vi "Find Icon With Most Depth.vi"(0 "Icon Info":T1[](array[typedef])=[{"Width"=16, "Height"=16, "Depth"=8, "Resource Data"=[40, 0, 0, 0, 16, 0, 0, 0, 32, 0, 0, 0, 1, 0, 8, 0, 0, 0, 0, 0, 64, 1, 0, 0, 0, 0, 0, 0, 0, 0, 0, 0, 0, 0, 0, 0, 0, 0, 0, 0, 0, 0, 0, 0, 128, 0, 128, 0, 128, 0, 0, 0, 146, 126, 107, 0, 0, 128, 0, 0, 0, 128, 128, 0, 0, 0, 128, 0, 188, 165, 151, 0, 191, 174, 160, 0, 233, 207, 188, 0, 154, 130, 111, 0, 255, 0, 255, 0, 255, 0, 0, 0, 255, 255, 0, 0, 0, 255, 0, 0, 0, 255, 255, 0, 0, 0, 255, 0, 255, 255, 255, 0, 224, 241, 253, 0, 187, 167, 153, 0, 225, 242, 253, 0, 193, 229, 254, 0, 132, 204, 253, 0, 119, 198, 252, 0, 69, 157, 219, 0, 10, 153, 252, 0, 10, 153, 251, 0, 19, 156, 252, 0, 0, 122, 185, 0, 0, 98, 150, 0, 0, 74, 115, 0, 0, 50, 80, 0, 193, 228, 253, 0, 159, 214, 253, 0, 121, 198, 253, 0, 97, 189, 252, 0, 52, 170, 252, 0, 41, 165, 252, 0, 24, 159, 252, 0, 0, 73, 220, 0, 0, 61, 185, 0, 0, 49, 150, 0, 0, 37, 115, 0, 0, 25, 80, 0, 156, 214, 253, 0, 117, 197, 252, 0, 102, 191, 253, 0, 55, 171, 252, 0, 67, 155, 216, 0, 37, 37, 255, 0, 0, 0, 255, 0, 0, 0, 220, 0, 0, 0, 185, 0, 0, 0, 150, 0, 0, 0, 115, 0, 0, 0, 80, 0, 156, 213, 253, 0, 132, 203, 252, 0, 91, 186, 252, 0, 132, 202, 252, 0, 115, 72, 255, 0, 87, 37, 255, 0, 85, 0, 255, 0, 73, 0, 220, 0, 61, 0, 185, 0, 49, 0, 150, 0, 37, 0, 115, 0, 25, 0, 80, 0, 254, 252, 252, 0, 131, 202, 251, 0, 251, 245, 242, 0, 249, 242, 236, 0, 249, 241, 236, 0, 170, 37, 255, 0, 170, 0, 255, 0, 146, 0, 220, 0, 122, 0, 185, 0, 98, 0, 150, 0, 74, 0, 115, 0, 50, 0, 80, 0, 255, 254, 254, 0, 252, 248, 246, 0, 252, 246, 243, 0, 251, 244, 240, 0, 251, 245, 241, 0, 251, 244, 241, 0, 255, 0, 255, 0, 244, 229, 221, 0, 185, 0, 185, 0, 150, 0, 150, 0, 115, 0, 115, 0, 80, 0, 80, 0, 254, 252, 251, 0, 253, 249, 247, 0, 254, 251, 249, 0, 251, 244, 239, 0, 232, 208, 192, 0, 240, 223, 212, 0, 234, 212, 199, 0, 220, 0, 146, 0, 180, 157, 140, 0, 150, 0, 98, 0, 115, 0, 74, 0, 80, 0, 50, 0, 245, 236, 229, 0, 237, 220, 209, 0, 182, 159, 143, 0, 180, 157, 141, 0, 237, 216, 204, 0, 255, 37, 87, 0, 255, 0, 85, 0, 220, 0, 73, 0, 185, 0, 61, 0, 150, 0, 49, 0, 115, 0, 37, 0, 80, 0, 25, 0, 243, 231, 223, 0, 185, 168, 154, 0, 180, 156, 140, 0, 231, 207, 192, 0, 255, 72, 72, 0, 255, 37, 37, 0, 255, 0, 0, 0, 220, 0, 0, 0, 185, 0, 0, 0, 150, 0, 0, 0, 115, 0, 0, 0, 80, 0, 0, 0, 253, 250, 248, 0, 252, 248, 244, 0, 181, 157, 142, 0, 181, 158, 142, 0, 235, 214, 201, 0, 255, 87, 37, 0, 255, 85, 0, 0, 220, 73, 0, 0, 185, 61, 0, 0, 150, 49, 0, 0, 115, 37, 0, 0, 80, 25, 0, 0, 250, 241, 235, 0, 252, 248, 245, 0, 235, 216, 203, 0, 233, 212, 197, 0, 251, 243, 239, 0, 238, 219, 208, 0, 233, 211, 196, 0, 220, 146, 0, 0, 172, 150, 134, 0, 150, 98, 0, 0, 115, 74, 0, 0, 80, 50, 0, 0, 254, 254, 253, 0, 253, 250, 249, 0, 252, 249, 246, 0, 252, 247, 245, 0, 251, 245, 240, 0, 251, 246, 243, 0, 255, 255, 0, 0, 241, 226, 217, 0, 222, 191, 171, 0, 179, 155, 139, 0, 134, 115, 95, 0, 80, 80, 0, 0, 253, 252, 250, 0, 252, 247, 244, 0, 252, 246, 244, 0, 232, 208, 193, 0, 250, 242, 238, 0, 170, 255, 37, 0, 170, 255, 0, 0, 146, 220, 0, 0, 122, 185, 0, 0, 98, 150, 0, 0, 74, 115, 0, 0, 50, 80, 0, 0, 253, 251, 250, 0, 251, 246, 242, 0, 184, 167, 152, 0, 250, 241, 236, 0, 115, 255, 72, 0, 87, 255, 37, 0, 85, 255, 0, 0, 73, 220, 0, 0, 61, 185, 0, 0, 49, 150, 0, 0, 37, 115, 0, 0, 25, 80, 0, 0, 253, 250, 247, 0, 252, 246, 242, 0, 180, 157, 139, 0, 232, 208, 194, 0, 72, 255, 72, 0, 37, 255, 37, 0, 0, 255, 0, 0, 0, 220, 0, 0, 0, 185, 0, 0, 0, 150, 0, 0, 0, 115, 0, 0, 0, 80, 0, 0, 222, 241, 254, 0, 192, 226, 249, 0, 250, 243, 238, 0, 249, 240, 235, 0, 72, 255, 115, 0, 37, 255, 87, 0, 0, 255, 85, 0, 0, 220, 73, 0, 0, 185, 61, 0, 0, 150, 49, 0, 0, 115, 37, 0, 0, 80, 25, 0, 253, 251, 249, 0, 132, 202, 251, 0, 138, 206, 253, 0, 251, 242, 238, 0, 250, 242, 236, 0, 37, 255, 170, 0, 0, 255, 170, 0, 0, 220, 146, 0, 0, 185, 122, 0, 0, 150, 98, 0, 0, 115, 74, 0, 0, 80, 50, 0, 254, 253, 252, 0, 140, 207, 253, 0, 143, 208, 253, 0, 108, 193, 252, 0, 65, 175, 252, 0, 30, 161, 252, 0, 0, 255, 255, 0, 39, 164, 252, 0, 0, 185, 185, 0, 0, 150, 150, 0, 0, 115, 115, 0, 0, 80, 80, 0, 252, 242, 237, 0, 236, 229, 226, 0, 241, 226, 216, 0, 217, 205, 197, 0, 193, 173, 158, 0, 185, 164, 149, 0, 187, 168, 154, 0, 186, 166, 151, 0, 184, 162, 147, 0, 182, 160, 144, 0, 156, 134, 115, 0, 133, 108, 86, 0, 128, 109, 89, 0, 160, 139, 121, 0, 74, 74, 74, 0, 62, 62, 62, 0, 50, 50, 50, 0, 38, 38, 38, 0, 26, 26, 26, 0, 14, 14, 14, 0, 0, 0, 0, 0, 100, 148, 249, 3, 162, 248, 248, 248, 248, 248, 248, 0, 0, 0, 0, 190, 72, 87, 159, 97, 145, 108, 132, 98, 146, 191, 160, 248, 0, 0, 0, 190, 81, 165, 157, 70, 85, 144, 168, 216, 179, 203, 119, 248, 0, 0, 0, 107, 93, 93, 141, 82, 177, 84, 83, 202, 215, 71, 96, 248, 0, 0, 0, 131, 94, 128, 93, 141, 165, 82, 70, 156, 95, 202, 167, 248, 0, 0, 0, 106, 92, 164, 94, 128, 93, 155, 166, 189, 70, 83, 143, 248, 26, 26, 26, 26, 26, 26, 26, 26, 26, 188, 154, 129, 82, 177, 142, 248, 26, 25, 25, 25, 25, 25, 25, 25, 26, 153, 128, 93, 141, 165, 105, 248, 26, 25, 231, 200, 47, 25, 26, 20, 26, 92, 176, 153, 188, 81, 238, 248, 26, 25, 225, 32, 56, 25, 26, 20, 26, 224, 68, 164, 212, 128, 116, 248, 26, 27, 20, 229, 18, 38, 26, 20, 26, 80, 152, 224, 92, 164, 104, 248, 26, 227, 33, 25, 226, 45, 26, 20, 26, 17, 17, 237, 8, 117, 178, 248, 26, 20, 36, 25, 37, 20, 26, 20, 26, 17, 17, 239, 140, 9, 247, 0, 26, 25, 25, 25, 25, 25, 25, 25, 26, 17, 17, 239, 236, 246, 0, 0, 26, 26, 26, 26, 26, 26, 26, 26, 26, 17, 17, 239, 240, 0, 0, 0, 0, 0, 0, 0, 242, 19, 243, 241, 244, 245, 130, 118, 0, 0, 0, 0, 240, 1, 255, 255, 224, 0, 255, 255, 224, 0, 255, 255, 224, 0, 255, 255, 224, 0, 255, 255, 224, 0, 255, 255, 0, 0, 255, 255, 0, 0, 255, 255, 0, 0, 255, 255, 0, 0, 255, 255, 0, 0, 255, 255, 0, 0, 255, 255, 0, 1, 255, 255, 0, 3, 255, 255, 0, 7, 255, 255, 240, 15, 255, 255]}, ...(7 in all)], 1 "Icon Size [px] (16)":u8=16) -> (2 "Icon Index":i32)   [LabVIEW 2019, in "VIPM.lvlib" / "VIPM Item.lvclass"]
uses:
  VIPM Item.lvclass
  <vilib>/Platform/icon.llb/IconInfo.ctl
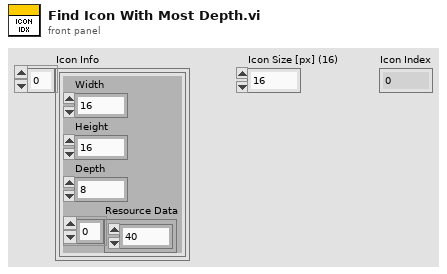
[diagram p1: front panel]
types:
  T1 = typedef "IconInfo.ctl" = cluster{"Width":u8, "Height":u8, "Depth":u8, "Resource Data":u8[]}
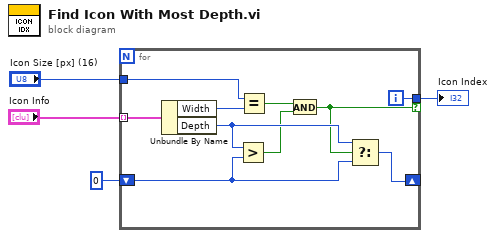
[diagram p0: block diagram]
diagram:
  n1 = for {
    tunnel: "Icon Info" -> [w14] mode=indexing
    shift-right: [w11] -> _
    shift-left: u8 0 ("Depth") -> [w10]
    tunnel: [w7] -> w2 if=w6
    tunnel: "Icon Size [px] (16)" -> [w5]
    i -> [w7]
    n2 = Unbundle By Name(w14) -> ("Width"=w13:u8, "Depth"=w12:u8)
    n3 = Greater?(x=w12, y=w10) -> (0:w8:bool)
    n4 = Equal?(x=w5, y=w13) -> (x = y?=w9:bool)
    n5 = And(x=w9, y=w8) -> (x .and. y?=w6:bool)
    n6 = Select(t=w12, s=w6, f=w10) -> (s? t:f=w11:u8)
  }
  "Icon Index" <- w2
